vi "niDTS WLAN Dut Tx Initiate.vi"(0 "Dut Handle in":T1, 11 "error in (no error)":errorcluster) -> (4 "Dut Handle out":T1, 15 "error out":errorcluster)   [LabVIEW 2015, in "niDTS WLAN.lvlib"]
uses:
  niDTS WLAN.lvlib
  Framework/Dut/Includes/niDTS Dut INC Handle.ctl
  Framework/Dut/Objects/BASE_class/niDTS Dut.lvclass
  Includes/niDTS WLAN Dut INC Handle.ctl
  Objects/BASE_class/niDTS WLAN Dut.lvclass
  Framework/niDTS Framework.lvlib
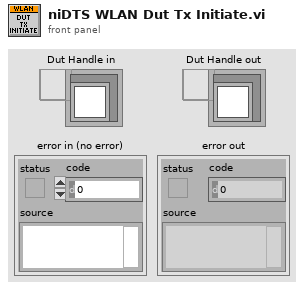
[diagram p1: front panel]
types:
  T1 = typedef "niDTS Framework.lvlib/niDTS Dut INC Handle.ctl" = refnum<data-value>
  T2 = typedef "niDTS WLAN.lvlib/niDTS WLAN Dut INC Handle.ctl" = refnum<data-value>
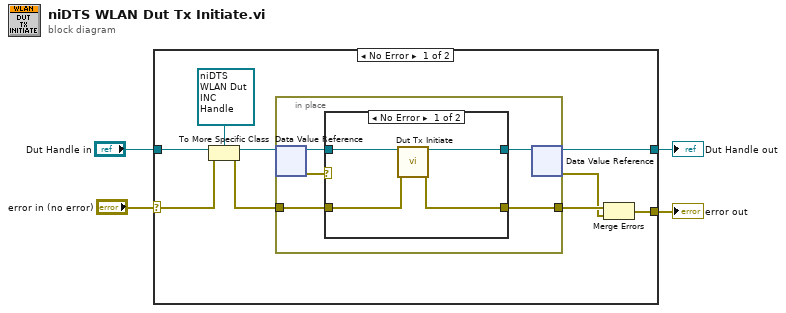
[diagram p0: block diagram]
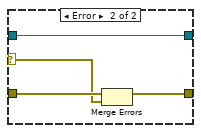
[diagram p2: hidden frame]
diagram:
  n1 = case shown="No Error" "error in (no error)" {
    selector: "error in (no error)" -> [w8 w27]
    tunnel: [w13 w28] -> w4
    tunnel: [w5 w27] -> w3
    tunnel: "Dut Handle in" -> [w11 w28]
    frame No Error {
      n2 = To More Specific Class(target class=T2 refnum ("WLAN Dut Handle"), reference=w11, error in=w8) -> (specific class reference=w10:T2, error out=w9:errorcluster)
      n3 = in-place {
        in-place-border: w9 -> [w15]
        in-place-border: [w14] -> w7
        n4 = in-place-dvr #1(w10) -> (w17:refnum<class "niDTS WLAN Dut.lvclass">, w18:errorcluster)
        n5 = case shown="No Error" w18 {
          selector: w18 -> [_ w24]
          tunnel: w17 -> [w22 w26]
          tunnel: [w21 w26] -> w16
          tunnel: w15 -> [w20 w25]
          tunnel: [w19 w23] -> w14
          frame No Error {
            n6 = call-dynamic "Dut Tx Initiate.vi"("niDTS DUT in"=w22, "error in (no error)"=w20) -> ("niDTS DUT out"=w21:refnum<class "niDTS WLAN Dut.lvclass">, "error out"=w19:errorcluster)  [unwired: 12 in]
          }
          frame Error {
            n7 = Merge Errors(w25, w24) -> (w23:errorcluster)
          }
        }
        n8 = in-place-dvr #1(w16) -> (w13:T2, w6:errorcluster)
      }
      n9 = Merge Errors(w7, w6) -> (w5:errorcluster)
    }
    frame Error {
    }
  }
  "Dut Handle out" <- w4
  "error out" <- w3
